vi "Default Colors.vi"(11 "Index":i32) -> (3 "Color":u32(colorbox))   [LabVIEW 2015, in "SB SubVIs.lvlib"]
uses:
  SB SubVIs.lvlib
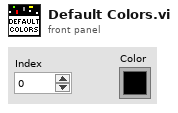
[diagram p1: front panel]
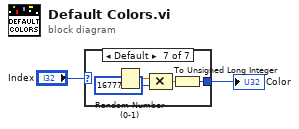
[diagram p0: block diagram]
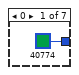
[diagram p2: hidden frame]
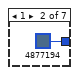
[diagram p3: hidden frame]
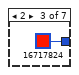
[diagram p4: hidden frame]
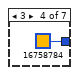
[diagram p5: hidden frame]
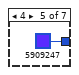
[diagram p6: hidden frame]
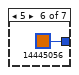
[diagram p7: hidden frame]
diagram:
  n1 = case shown="Default" "Index" {
    tunnel: [u32 40774 u32 4877194 u32 16717824 u32 16758784 u32 5909247 u32 14445056 w10] -> w1
    frame 0 {
    }
    frame 1 {
    }
    frame 2 {
    }
    frame 3 {
    }
    frame 4 {
    }
    frame 5 {
    }
    frame Default {
      n2 = Random Number (0-1)() -> (number: 0 to 1=w9:dbl)
      n3 = Compound Arithmetic op=MULTIPLY(w9, 16777215) -> (w12:dbl)
      n4 = To Unsigned Long Integer(number=w12) -> (unsigned 32bit integer=w10:u32)
    }
  }
  "Color" <- w1
